vi "DS18B20 - convert raw temp.vi"(11 "Raw Temp":u16) -> (2 "Temp (F)":sgl, 3 "Temp (C)":sgl)   [LabVIEW 2013]
panel:
  in  "test":bool
  in  "MSB":u8 format="%.0x"
  in  "LSB":u8 format="%.0x"
  # "Perform the temperature conversion for DS18B20\n- takes the raw 16 bit data coming from FPGA or LSB and MSB depending on boolean\n- calculates temperature in C and F"
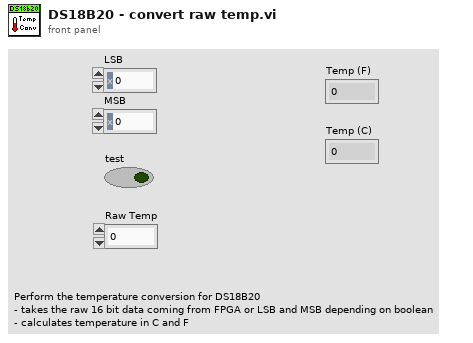
[diagram p1: front panel]
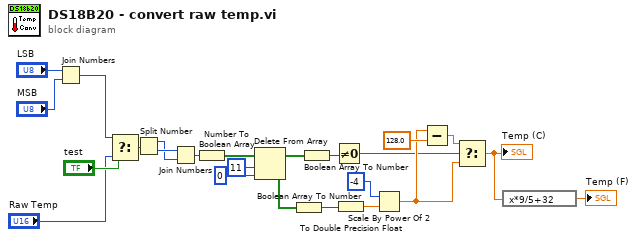
[diagram p0: block diagram]
diagram:
  n1 = Join Numbers(hi="LSB", lo="MSB") -> ((hi.lo)=w2:u16)
  n2 = Select(t=w2, s="test", f="Raw Temp") -> (s? t:f=w4:u16)
  n3 = Split Number(x=w4) -> (hi(x)=w21:u8, lo(x)=w22:u8)
  n4 = Join Numbers(hi=w22, lo=w21) -> ((hi.lo)=w20:u16)
  n5 = Number To Boolean Array(number=w20) -> (Boolean array=w19:bool[])
  n6 = Delete From Array(array=w19, length=11, index=0) -> (deleted portion=w16:bool[], array with subset deleted=w11:bool[])
  n7 = Boolean Array To Number(Boolean array=w16) -> (number=w13:u16)
  n8 = Boolean Array To Number(Boolean array=w11) -> (number=w10:u8)
  n9 = Not Equal To 0?(x=w10) -> (x != 0?=w9:bool)
  n10 = To Double Precision Float(number=w13) -> (double precision float=w14:dbl)
  n11 = Scale By Power Of 2(n=-4, x=w14) -> (x*2^n=w12:dbl)
  n12 = Subtract(x=w12, y=128.0 ("x")) -> (x-y=w24:dbl)
  n13 = Select(t=w24, s=w9, f=w12) -> (s? t:f=w8:dbl)
  "Temp (C)" <- w8
  n14 = expression code="x*9/5+32"(w8) -> (→"Temp (F)":dbl)
